vi "ex_Loundry_Machine.vi"() -> ()   [LabVIEW 2022 SP3]
doc: "This is the VI which is a simple Loundry Machine"
uses:
  #typedef_Wanding_machine_task.ctl
  #typedef_Wanding_machine_operation.ctl
  #typedef_Wanding_machine_states.ctl
  Traffic_Lights/#typedef_TimerAction.ctl
  #typedef_Wanding_machine_programdata.ctl
panel:
  out "Kind of Operation":T1
  in  "Dial":T2 scale=0.0..4.0
  in  "Lid Open":bool
  in  "Drying Enable":bool
  in  "Start":bool
  in  "stop":bool
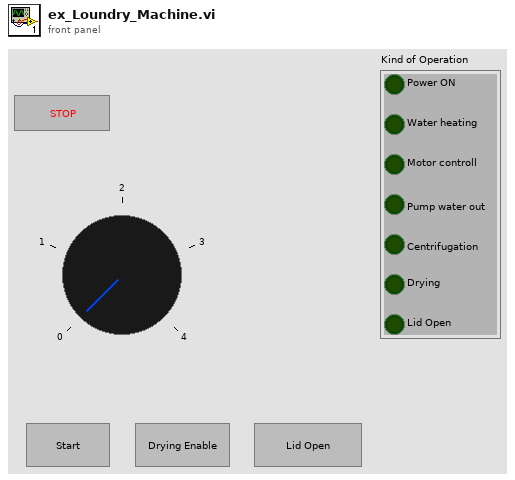
[diagram p1: front panel]
types:
  T1 = typedef "#typedef_Wanding_machine_operation.ctl" = cluster{"Power ON":bool, "Water heating":bool, "Motor controll":bool, "Pump water out ":bool, "Centrifugation":bool, "Drying":bool, "Lid Open":bool}
  T2 = typedef "#typedef_Wanding_machine_task.ctl" = i32
  T3 = typedef "#typedef_Wanding_machine_states.ctl" = enum16{"Drying (Led On)", "Water Heating", "Wait For Event", "Initialize", "Error Handler", "Exit", "Centrifugation", "Pump Water Out", "Drying", "Motor Controll"}
  T4 = typedef "#typedef_TimerAction.ctl" = enum16{"Reset", "TimeElapsed"}
  T5 = typedef "#typedef_Wanding_machine_programdata.ctl" = cluster{"Kind Of Operation":T1, "Task":T2}
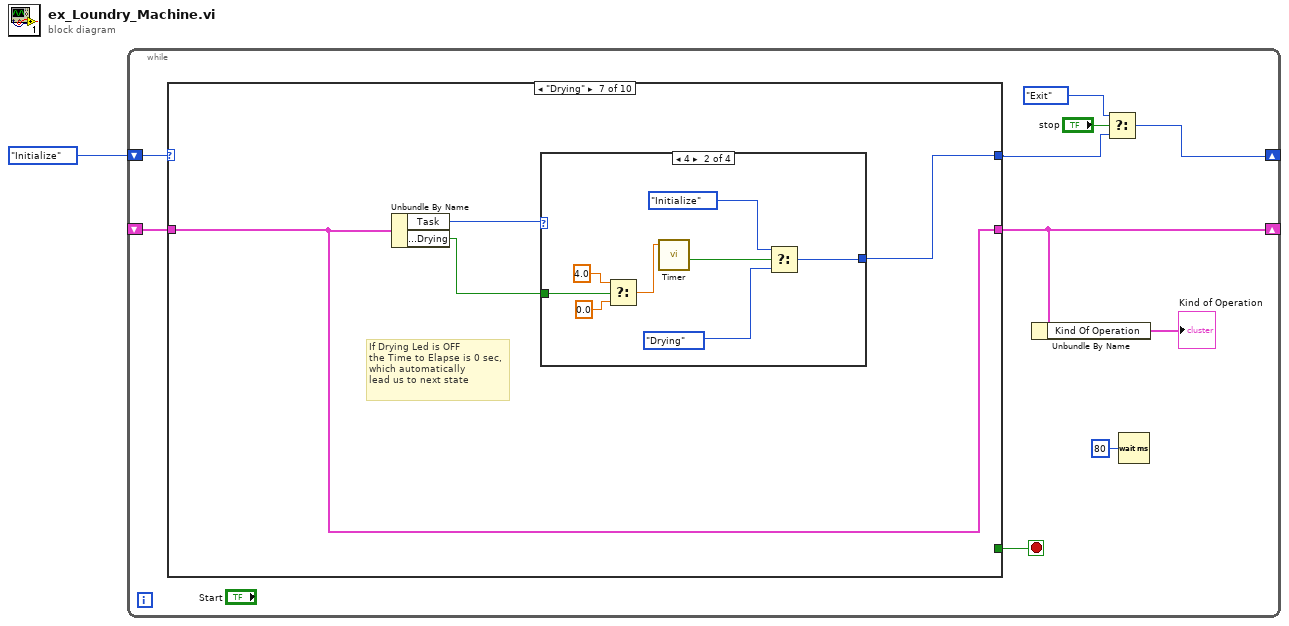
[diagram p0: block diagram]
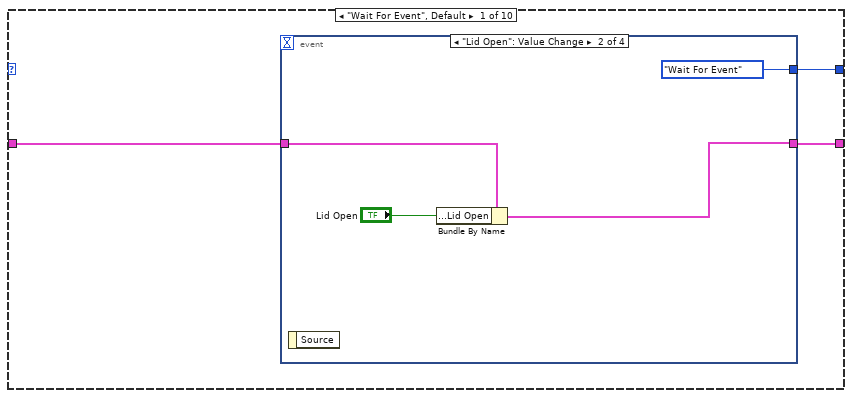
[diagram p2: hidden frame]
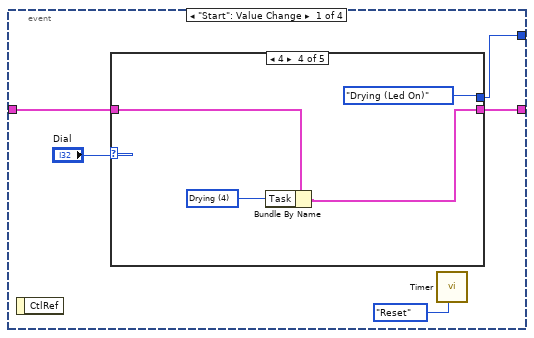
[diagram p3: hidden frame]
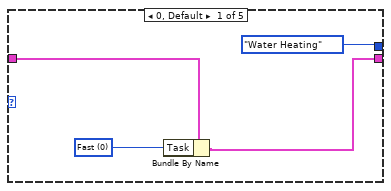
[diagram p4: hidden frame]
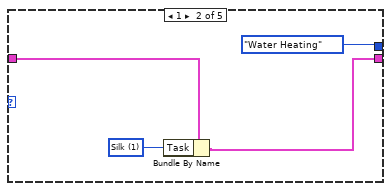
[diagram p5: hidden frame]
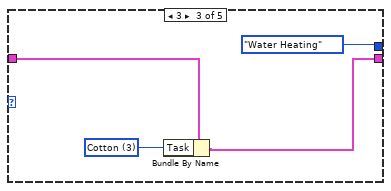
[diagram p6: hidden frame]
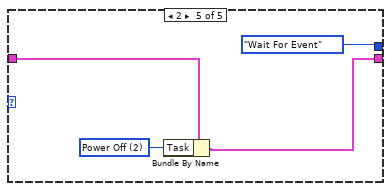
[diagram p7: hidden frame]
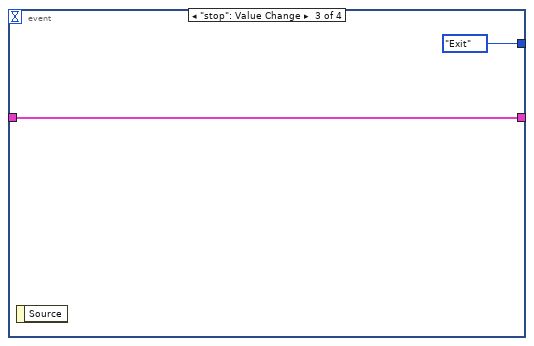
[diagram p8: hidden frame]
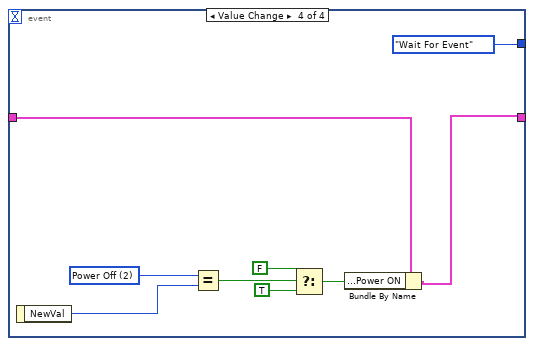
[diagram p9: hidden frame]
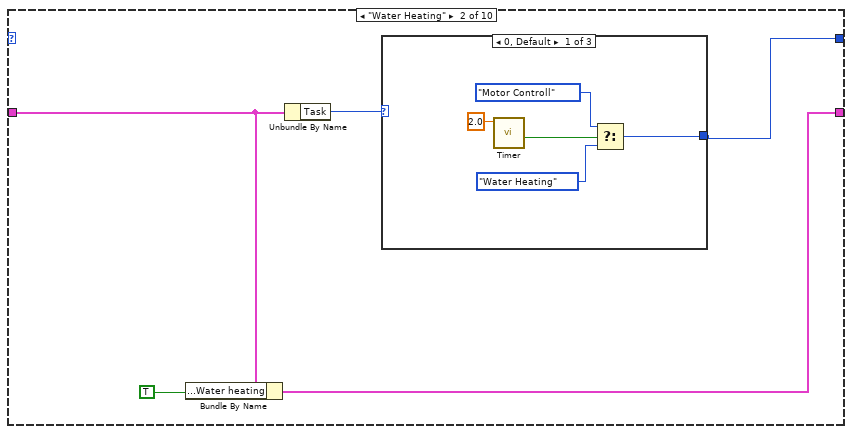
[diagram p10: hidden frame]
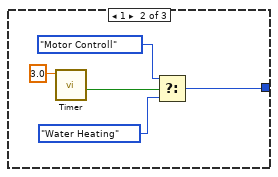
[diagram p11: hidden frame]
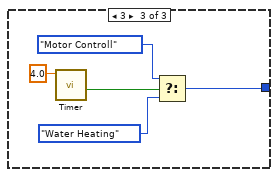
[diagram p12: hidden frame]
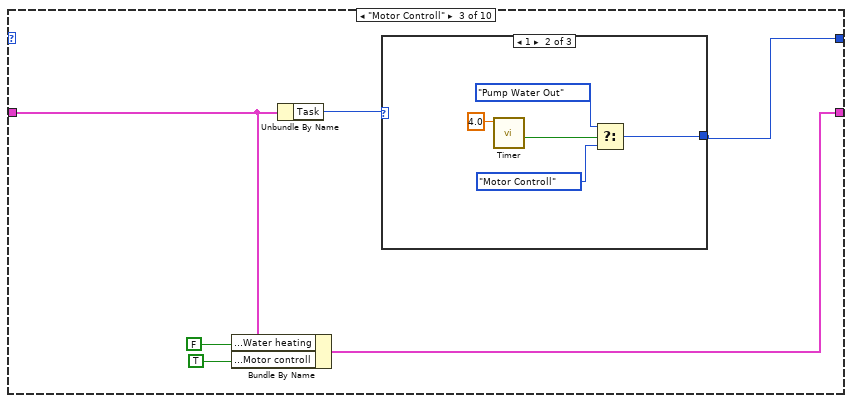
[diagram p13: hidden frame]
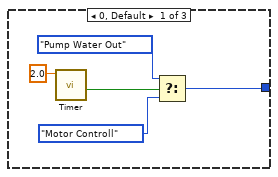
[diagram p14: hidden frame]
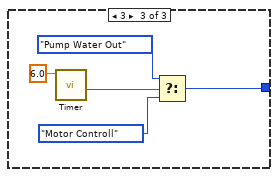
[diagram p15: hidden frame]
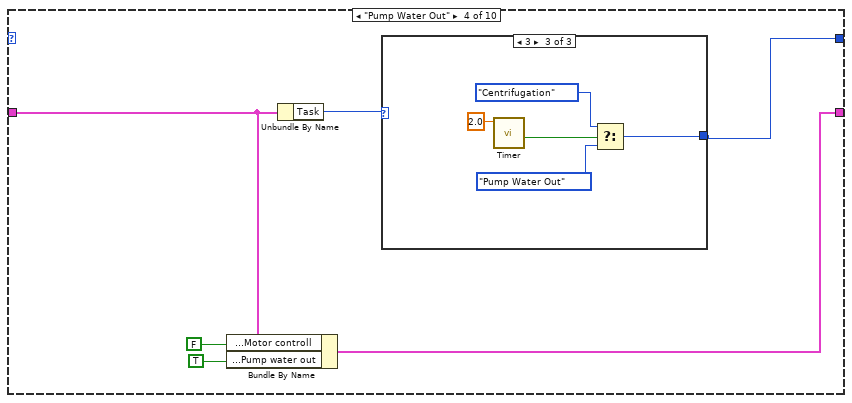
[diagram p16: hidden frame]
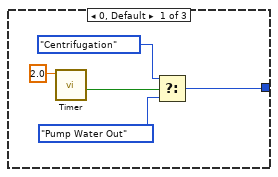
[diagram p17: hidden frame]
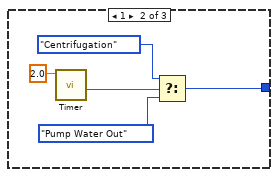
[diagram p18: hidden frame]
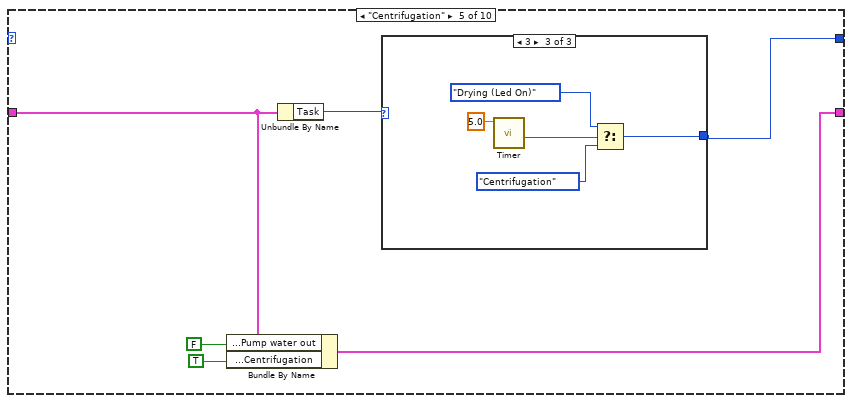
[diagram p19: hidden frame]
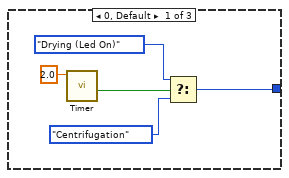
[diagram p20: hidden frame]
diagram:
  n1 = while {
    shift-right: [w6] -> _
    shift-left: #typedef_Wanding_machine_states."Initialize" ("SM_States") -> [w11]
    shift-right: [w4] -> _
    shift-left: _ -> [w10]
    stop <- w5 stop-if-true
    n2 = case shown="\"Drying\"" w11 {
      tunnel: [w12 w55 w78 w99 w120 w140 w143 T5 {"Kind Of Operation"={"Power ON"=TRUE, "Water heating"=FALSE, "Motor controll"=FALSE, "Pump water out "=FALSE, "Centrifugation"=FALSE, "Drying"=FALSE, "Lid Open"=FALSE}, "Task"=0} ("Wanding_Machine_programData") w182 w186] -> w4
      tunnel: [w14 w58 w76 w97 w118 #typedef_Wanding_machine_states."Drying" ("t") w145 #typedef_Wanding_machine_states."Wait For Event" ("SM_States") #typedef_Wanding_machine_states."Exit" ("t") #typedef_Wanding_machine_states."Exit" ("t")] -> w8
      tunnel: w10 -> [w13 w56 w80 w101 w122 w142 w143 _ w182 w186]
      tunnel: [_ _ _ _ _ _ _ _ TRUE w188] -> w5
      frame "Wait For Event", Default {
        n3 = event shown="[1] \"Lid Open\": Value Change" {
          selector: _ -> [_ _ _ _]
          dyn-events: _ -> [_ _ _ _]
          timeout: _ -> [_ _ _ _]
          tunnel: [w18 #typedef_Wanding_machine_states."Wait For Event" ("SM_States") #typedef_Wanding_machine_states."Exit" ("t") #typedef_Wanding_machine_states."Wait For Event" ("t")] -> w14
          tunnel: w13 -> [w17 w42 w44 w51]
          tunnel: [w16 w41 w44 w47] -> w12
          event "Start": Value Change {
            n4 = event-data() -> ()  [unwired: 1 in, 1 out]
            n5 = case shown="4" "Dial" {
              tunnel: [#typedef_Wanding_machine_states."Water Heating" ("SM_States") #typedef_Wanding_machine_states."Water Heating" ("SM_States") #typedef_Wanding_machine_states."Water Heating" ("SM_States") #typedef_Wanding_machine_states."Drying (Led On)" ("SM_States") #typedef_Wanding_machine_states."Wait For Event" ("SM_States")] -> w18
              tunnel: w17 -> [w22 w26 w30 w34 w38]
              tunnel: [w20 w24 w28 w32 w36] -> w16
              frame 0, Default {
                w21 = T2 0 items=["Fast", "Silk", "Power Off", "Cotton", "Drying"] ("Task")
                n6 = Bundle By Name(cluster=w22, "Task"=w21) -> (w20:T5)
              }
              frame 1 {
                w25 = T2 1 items=["Fast", "Silk", "Power Off", "Cotton", "Drying"] ("Task")
                n7 = Bundle By Name(cluster=w26, "Task"=w25) -> (w24:T5)
              }
              frame 3 {
                w29 = T2 3 items=["Fast", "Silk", "Power Off", "Cotton", "Drying"] ("Task")
                n8 = Bundle By Name(cluster=w30, "Task"=w29) -> (w28:T5)
              }
              frame 4 {
                w33 = T2 4 items=["Fast", "Silk", "Power Off", "Cotton", "Drying"] ("Task")
                n9 = Bundle By Name(cluster=w34, "Task"=w33) -> (w32:T5)
              }
              frame 2 {
                w37 = T2 2 items=["Fast", "Silk", "Power Off", "Cotton", "Drying"] ("Task")
                n10 = Bundle By Name(cluster=w38, "Task"=w37) -> (w36:T5)
              }
            }
            n11 = call "Timer.vi"("Action (Time Elapsed)"=#typedef_TimerAction."Reset") -> ()  [unwired: 8 in, 3 out]
          }
          event "Lid Open": Value Change {
            n12 = event-data() -> ()  [unwired: 1 in, 1 out]
            n13 = Bundle By Name(cluster=w42, "Kind Of Operation.Lid Open"="Lid Open") -> (w41:T5)
          }
          event "stop": Value Change {
            n14 = event-data() -> ()  [unwired: 1 in, 1 out]
          }
          event Value Change {
            w53 = T2 2 items=["Fast", "Silk", "Power Off", "Cotton", "Drying"] ("x")
            n15 = event-data() -> ("NewVal"=w54:T2)  [unwired: 1 in]
            n16 = Equal?(x=w53, y=w54) -> (x = y?=w52:bool)
            n17 = Select(t=FALSE, s=w52, f=TRUE) -> (s? t:f=w48:bool)
            n18 = Bundle By Name(cluster=w51, "Kind Of Operation.Power ON"=w48) -> (w47:T5)
          }
        }
      }
      frame "Water Heating" {
        n19 = Bundle By Name(cluster=w56, "Kind Of Operation.Water heating"=TRUE) -> (w55:T5)
        n20 = Unbundle By Name(w56) -> ("Task"=w59:T2)
        n21 = case shown="0, Default" w59 {
          tunnel: [w60 w65 w70] -> w58
          frame 0, Default {
            n22 = call "Timer.vi"("Time To Elapse"=2.0) -> ("Time Elapsed?"=w63:bool)  [unwired: 8 in, 2 out]
            n23 = Select(t=#typedef_Wanding_machine_states."Motor Controll" ("SM_States"), s=w63, f=#typedef_Wanding_machine_states."Water Heating" ("SM_States")) -> (s? t:f=w60:T3)
          }
          frame 1 {
            n24 = call "Timer.vi"("Time To Elapse"=3.0) -> ("Time Elapsed?"=w68:bool)  [unwired: 8 in, 2 out]
            n25 = Select(t=#typedef_Wanding_machine_states."Motor Controll" ("SM_States"), s=w68, f=#typedef_Wanding_machine_states."Water Heating" ("SM_States")) -> (s? t:f=w65:T3)
          }
          frame 3 {
            n26 = call "Timer.vi"("Time To Elapse"=4.0) -> ("Time Elapsed?"=w73:bool)  [unwired: 8 in, 2 out]
            n27 = Select(t=#typedef_Wanding_machine_states."Motor Controll" ("SM_States"), s=w73, f=#typedef_Wanding_machine_states."Water Heating" ("SM_States")) -> (s? t:f=w70:T3)
          }
        }
      }
      frame "Motor Controll" {
        n28 = Bundle By Name(cluster=w80, "Kind Of Operation.Water heating"=FALSE, "Kind Of Operation.Motor controll"=TRUE) -> (w78:T5)
        n29 = Unbundle By Name(w80) -> ("Task"=w77:T2)
        n30 = case shown="1" w77 {
          tunnel: [w81 w86 w91] -> w76
          frame 0, Default {
            n31 = call "Timer.vi"("Time To Elapse"=2.0) -> ("Time Elapsed?"=w84:bool)  [unwired: 8 in, 2 out]
            n32 = Select(t=#typedef_Wanding_machine_states."Pump Water Out" ("SM_States"), s=w84, f=#typedef_Wanding_machine_states."Motor Controll" ("SM_States")) -> (s? t:f=w81:T3)
          }
          frame 1 {
            n33 = call "Timer.vi"("Time To Elapse"=4.0) -> ("Time Elapsed?"=w89:bool)  [unwired: 8 in, 2 out]
            n34 = Select(t=#typedef_Wanding_machine_states."Pump Water Out" ("SM_States"), s=w89, f=#typedef_Wanding_machine_states."Motor Controll" ("SM_States")) -> (s? t:f=w86:T3)
          }
          frame 3 {
            n35 = call "Timer.vi"("Time To Elapse"=6.0) -> ("Time Elapsed?"=w94:bool)  [unwired: 8 in, 2 out]
            n36 = Select(t=#typedef_Wanding_machine_states."Pump Water Out" ("SM_States"), s=w94, f=#typedef_Wanding_machine_states."Motor Controll" ("SM_States")) -> (s? t:f=w91:T3)
          }
        }
      }
      frame "Pump Water Out" {
        n37 = Bundle By Name(cluster=w101, "Kind Of Operation.Motor controll"=FALSE ("Kind Of Operation.Water heating"), "Kind Of Operation.Pump water out"=TRUE ("Kind Of Operation.Motor controll")) -> (w99:T5)
        n38 = Unbundle By Name(w101) -> ("Task"=w98:T2)
        n39 = case shown="3" w98 {
          tunnel: [w102 w107 w112] -> w97
          frame 0, Default {
            n40 = call "Timer.vi"("Time To Elapse"=2.0) -> ("Time Elapsed?"=w105:bool)  [unwired: 8 in, 2 out]
            n41 = Select(t=#typedef_Wanding_machine_states."Centrifugation" ("SM_States"), s=w105, f=#typedef_Wanding_machine_states."Pump Water Out" ("SM_States")) -> (s? t:f=w102:T3)
          }
          frame 1 {
            n42 = call "Timer.vi"("Time To Elapse"=2.0) -> ("Time Elapsed?"=w110:bool)  [unwired: 8 in, 2 out]
            n43 = Select(t=#typedef_Wanding_machine_states."Centrifugation" ("SM_States"), s=w110, f=#typedef_Wanding_machine_states."Pump Water Out" ("SM_States")) -> (s? t:f=w107:T3)
          }
          frame 3 {
            n44 = call "Timer.vi"("Time To Elapse"=2.0) -> ("Time Elapsed?"=w115:bool)  [unwired: 8 in, 2 out]
            n45 = Select(t=#typedef_Wanding_machine_states."Centrifugation" ("SM_States"), s=w115, f=#typedef_Wanding_machine_states."Pump Water Out" ("SM_States")) -> (s? t:f=w112:T3)
          }
        }
      }
      frame "Centrifugation" {
        n46 = Bundle By Name(cluster=w122, "Kind Of Operation.Pump water out"=FALSE ("Kind Of Operation.Water heating"), "Kind Of Operation.Centrifugation"=TRUE ("Kind Of Operation.Motor controll")) -> (w120:T5)
        n47 = Unbundle By Name(w122) -> ("Task"=w119:T2)
        n48 = case shown="3" w119 {
          tunnel: [w123 w128 w133] -> w118
          frame 0, Default {
            n49 = call "Timer.vi"("Time To Elapse"=2.0) -> ("Time Elapsed?"=w126:bool)  [unwired: 8 in, 2 out]
            n50 = Select(t=#typedef_Wanding_machine_states."Drying (Led On)" ("SM_States"), s=w126, f=#typedef_Wanding_machine_states."Centrifugation" ("SM_States")) -> (s? t:f=w123:T3)
          }
          frame 1 {
            n51 = call "Timer.vi"("Time To Elapse"=3.0) -> ("Time Elapsed?"=w131:bool)  [unwired: 8 in, 2 out]
            n52 = Select(t=#typedef_Wanding_machine_states."Drying (Led On)" ("SM_States"), s=w131, f=#typedef_Wanding_machine_states."Centrifugation" ("SM_States")) -> (s? t:f=w128:T3)
          }
          frame 3 {
            n53 = call "Timer.vi"("Time To Elapse"=5.0) -> ("Time Elapsed?"=w136:bool)  [unwired: 8 in, 2 out]
            n54 = Select(t=#typedef_Wanding_machine_states."Drying (Led On)" ("SM_States"), s=w136, f=#typedef_Wanding_machine_states."Centrifugation" ("SM_States")) -> (s? t:f=w133:T3)
          }
        }
      }
      frame "Drying (Led On)" {
        n55 = Bundle By Name(cluster=w142, "Kind Of Operation.Drying"="Drying Enable", "Kind Of Operation.Centrifugation"=FALSE) -> (w140:T5)
      }
      frame "Drying" {
        # "If Drying Led is OFF\nthe Time to Elapse is 0 sec,\nwhich automatically \nlead us to next state"
        n56 = Unbundle By Name(w143) -> ("Task"=w146:T2, "Kind Of Operation.Drying"=w144:bool)
        n57 = case shown="4" w146 {
          tunnel: [w152 w160 w168 w176] -> w145
          tunnel: w144 -> [w149 w156 w167 w173]
          frame 3 {
            n58 = Select(t=5.0, s=w149, f=0.0) -> (s? t:f=w148:dbl)
            n59 = call "Timer.vi"("Time To Elapse"=w148) -> ("Time Elapsed?"=w147:bool)  [unwired: 8 in, 2 out]
            n60 = Select(t=#typedef_Wanding_machine_states."Initialize" ("SM_States"), s=w147, f=#typedef_Wanding_machine_states."Drying" ("SM_States")) -> (s? t:f=w152:T3)
          }
          frame 4 {
            n61 = Select(t=4.0, s=w156, f=0.0) -> (s? t:f=w155:dbl)
            n62 = call "Timer.vi"("Time To Elapse"=w155) -> ("Time Elapsed?"=w159:bool)  [unwired: 8 in, 2 out]
            n63 = Select(t=#typedef_Wanding_machine_states."Initialize" ("SM_States"), s=w159, f=#typedef_Wanding_machine_states."Drying" ("SM_States")) -> (s? t:f=w160:T3)
          }
          frame 0, Default {
            n64 = Select(t=2.0, s=w167, f=0.0) -> (s? t:f=w164:dbl)
            n65 = call "Timer.vi"("Time To Elapse"=w164) -> ("Time Elapsed?"=w163:bool)  [unwired: 8 in, 2 out]
            n66 = Select(t=#typedef_Wanding_machine_states."Initialize" ("SM_States"), s=w163, f=#typedef_Wanding_machine_states."Drying" ("SM_States")) -> (s? t:f=w168:T3)
          }
          frame 1 {
            n67 = Select(t=2.0, s=w173, f=0.0) -> (s? t:f=w172:dbl)
            n68 = call "Timer.vi"("Time To Elapse"=w172) -> ("Time Elapsed?"=w171:bool)  [unwired: 8 in, 2 out]
            n69 = Select(t=#typedef_Wanding_machine_states."Initialize" ("SM_States"), s=w171, f=#typedef_Wanding_machine_states."Drying" ("SM_States")) -> (s? t:f=w176:T3)
          }
        }
      }
      frame "Initialize" {
        n70 = call "Timer.vi"("Action (Time Elapsed)"=#typedef_TimerAction."Reset") -> ()  [unwired: 8 in, 3 out]
      }
      frame "Exit" {
      }
      frame "Error Handler" {
        n71 = One Button Dialog(message="Application Error") -> (true=w188:bool)  [unwired: 1 in]
      }
    }
    n72 = Unbundle By Name(w4) -> ("Kind Of Operation"=→"Kind of Operation":T1)
    n73 = Select(t=#typedef_Wanding_machine_states."Exit", s="stop", f=w8) -> (s? t:f=w6:T3)
    n74 = Wait (ms)(milliseconds to wait=u32 80) -> ()  [unwired: 1 out]
  }
